vi "MessageLogAnalyser.vi"() -> ()   [LabVIEW 2020]
panel:
  in  "folder Path":path
  in  "Template File":path=path "/Volumes/CentralDataCache/2021/GDW-Metadata/metadata/Logs/Logfile.tpt"
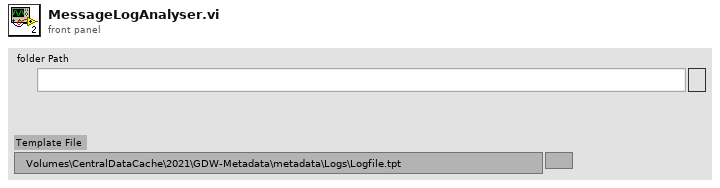
[diagram p1: front panel]
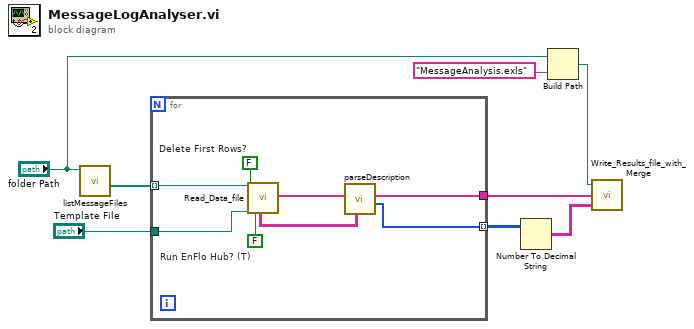
[diagram p0: block diagram]
diagram:
  n1 = call "listMessageFiles.vi"("folder Path"="folder Path") -> ("All Files in Dir"=w4:path[])  [unwired: 10 in]
  n2 = for {
    tunnel: "Template File" -> [w16]
    tunnel: [w11] -> w6
    tunnel: w4 -> [w10] mode=indexing
    tunnel: [w9] -> w7 mode=indexing
    w14 = FALSE  # Run EnFlo Hub? (T)
    w15 = FALSE  # Delete First Rows?
    n3 = call "Read_Data_file.vi"("Results file"=w10, "Delete First Rows?"=w15, "Template File"=w16, "Run EnFlo Hub? (T)"=w14) -> ("Deleted Rows"=w12:string[][], "Ch names Out"=w13:string[])  [unwired: 5 in, 9 out]
    n4 = call "parseDescription.vi"("Deleted Rows"=w12, "Ch names Out"=w13) -> ("values"=w9:i32[], "titles"=w11:string[])  [unwired: 8 in]
  }
  n5 = Number To Decimal String(number=w7) -> (decimal integer string=w5:string[][])  [unwired: 1 in]
  n6 = Build Path(base path="folder Path", name or relative path="MessageAnalysis.exls") -> (appended path=w2:path)
  n7 = call "Write_Results_file_with_Merge.vi"("Values In"=w5, "Channel Names in"=w6, "Filename"=w2) -> ()  [unwired: 1 in, 2 out]
